vi "Loop_End.vi"(1 "Position In":i32, 2 "Input Sequence":cluster{string, string[], dbl[], dbl}[](array[cluster]), 3 "Loop Count In":cluster{string, "Position":i32}[](array[cluster])) -> (0 "Position Out":i32)   [LabVIEW 2011]
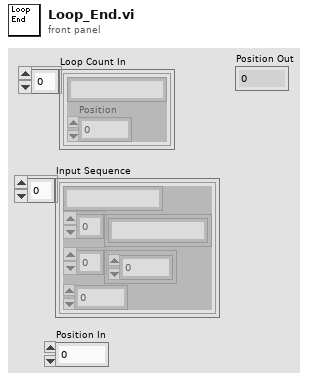
[diagram p1: front panel]
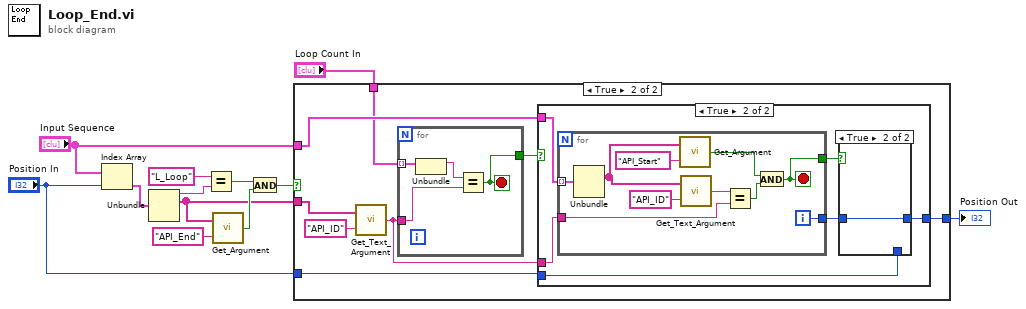
[diagram p0: block diagram]
diagram:
  n1 = Index Array(array="Input Sequence", index="Position In") -> (element=w5:cluster{string, string[], dbl[], dbl})
  n2 = Unbundle(w5) -> (w11:string, w3:string[])  [unwired: 2 out]
  n3 = Equal?(x="L_Loop", y=w11) -> (x = y?=w9:bool)
  n4 = call "Get_Argument.vi"("Argument"="API_End", "Argument List"=w3) -> ("Enabled"=w8:bool)
  n5 = And(x=w9, y=w8) -> (x .and. y?=w2:bool)
  n6 = case shown="True" w2 {
    tunnel: "Input Sequence" -> [_ w18]
    tunnel: w3 -> [_ w16]
    tunnel: [w13 w21] -> w7
    tunnel: "Position In" -> [w13 w20]
    tunnel: "Loop Count In" -> [_ w17]
    frame False {
    }
    frame True {
      n7 = call "Get_Text_Argument.vi"("Argument"="API_ID", "Argument List"=w16) -> ("Text"=w15:string)
      n8 = for {
        tunnel: w15 -> [w42]
        tunnel: [w43] -> w14
        tunnel: w17 -> [w41] mode=indexing
        stop <- w43 stop-if-true
        n9 = Unbundle(w41) -> (w44:string)  [unwired: 1 out]
        n10 = Equal?(x=w44, y=w42) -> (x = y?=w43:bool)
      }
      n11 = case shown="True" w14 {
        tunnel: [w22 w26] -> w21
        tunnel: w20 -> [w22 w25]
        tunnel: w18 -> [_ w24]
        tunnel: w15 -> [_ w23]
        frame False {
        }
        frame True {
          n12 = for {
            tunnel: w24 -> [w40] mode=indexing
            tunnel: w23 -> [w37]
            tunnel: [w32] -> w28
            tunnel: [w31] -> w27
            i -> [w31]
            stop <- w32 stop-if-true
            n13 = Unbundle(w40) -> (w36:string[])  [unwired: 3 out]
            n14 = call "Get_Argument.vi"("Argument"="API_Start", "Argument List"=w36) -> ("Enabled"=w33:bool)
            n15 = call "Get_Text_Argument.vi"("Argument"="API_ID", "Argument List"=w36) -> ("Text"=w38:string)
            n16 = Equal?(x=w38, y=w37) -> (x = y?=w34:bool)
            n17 = And(x=w33, y=w34) -> (x .and. y?=w32:bool)
          }
          n18 = case shown="True" w28 {
            tunnel: w27 -> [_ w30]
            tunnel: [w29 w30] -> w26
            tunnel: w25 -> [w29 _]
            frame False {
            }
            frame True {
            }
          }
        }
      }
    }
  }
  "Position Out" <- w7
